vi "pwm servo.vi"(4 "Control 5":dbl, 6 "Control 4":dbl, 7 "Control 6":dbl, 9 "Control 3":dbl, 10 "Control 2":dbl, 11 "Control 1":dbl) -> ()   [LabVIEW 2019]
uses:
  <vilib>/myRIO/Instrument Drivers/Onboard IO/PWM/typedefs/PWM Reference.ctl
  <vilib>/myRIO/Common/Instrument Driver Framework/Utilities/typedefs/myRIO Generic Hardware Reference.ctl
  <vilib>/myRIO/Common/Instrument Driver Framework/Utilities/typedefs/Hardware Version Enum.ctl
  <vilib>/myRIO/Common/Instrument Driver Framework/Utilities/typedefs/myRIO v1.0 Reference.ctl
  <vilib>/myRIO/Common/Instrument Driver Framework/Utilities/typedefs/Generic FPGA Reference.ctl
  <vilib>/myRIO/Common/Instrument Driver Framework/myRIO v1.0/PWM/typedefs/PWM Channels Enum.ctl
  <vilib>/myRIO/Instrument Drivers/Onboard IO/PWM/typedefs/PWM Configuration.ctl
  <vilib>/userdefined/High Color/nirio_resource_hc.ctl
  <vilib>/myRIO/Common/Instrument Driver Framework/Utilities/vis/Is FPGA Ref Available.vi
  <vilib>/myRIO/Common/Instrument Driver Framework/myRIO v1.0/PWM/vis/myRIO v1.1 Open PWM.vi
  <vilib>/myRIO/Instrument Drivers/Onboard IO/PWM/vis/Set Duty Cycle and Frequency.vi
  <vilib>/myRIO/Common/Instrument Driver Framework/Utilities/vis/Validate Channels.vi
  <vilib>/myRIO/Common/Instrument Driver Framework/myRIO v1.0/PWM/vis/myRIO v1.0 Reserve PWM.vi
  <vilib>/myRIO/Common/Instrument Driver Framework/myRIO v1.0/PWM/vis/myRIO v1.0 Build MUX Configuration PWM.vi
  <vilib>/myRIO/Common/Instrument Driver Framework/myRIO v1.0/Resource Manager/vis/myRIO v1.0 Reserve Channel List.vi
  <vilib>/myRIO/Common/Instrument Driver Framework/myRIO v1.0/Resource Manager/vis/myRIO v1.0 Create Configuration List.vi
  <vilib>/myRIO/Common/Instrument Driver Framework/myRIO v1.0/Resource Manager/vis/myRIO v1.0 Reserve Channel.vi
  <vilib>/myRIO/Common/Instrument Driver Framework/myRIO v1.0/Resource Manager/vis/myRIO v1.0 Unreserve Channel.vi
  <vilib>/myRIO/Common/Instrument Driver Framework/myRIO v1.0/Resource Manager/vis/myRIO v1.0 Build Mutex Name.vi
  <vilib>/Utility/VariantDataType/GetNumericInfo.vi
  <vilib>/Utility/error.llb/Error Cluster From Error Code.vi
  <vilib>/myRIO/Common/Instrument Driver Framework/myRIO v1.0/myRIO v1.1 Open.vi
  <vilib>/myRIO/Common/Instrument Driver Framework/Utilities/vis/IO Manager.vi
  <vilib>/myRIO/Common/Instrument Driver Framework/Utilities/vis/Configuration Manager.vi
  <vilib>/myRIO/Common/Instrument Driver Framework/myRIO v1.0/Resource Manager/vis/myRIO v1.0 Configure IO.vi
  <vilib>/myRIO/Common/Instrument Driver Framework/myRIO v1.0/myRIO v1.0 Close.vi
  <vilib>/myRIO/Common/Instrument Driver Framework/myRIO v1.0/PWM/vis/myRIO v1.0 Write PWM.vi
  <vilib>/myRIO/Express VI/Onboard IO/PWM/PWM Express VI.xnode
  <vilib>/myRIO/Instrument Drivers/Onboard IO/PWM/vis/myRIO PWM Open.xnode
  <vilib>/myRIO/Instrument Drivers/Onboard IO/PWM/PWM.lvlib
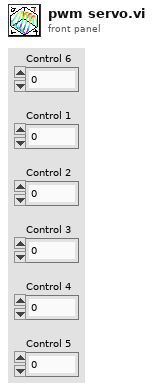
[diagram p1: front panel]
types:
  T1 = typedef "PWM.lvlib/PWM Reference.ctl" = cluster{"myRIO Reference":T2, "PWM Channels Enum":T6, "PWM Configuration":T7}
  T2 = typedef "myRIO Generic Hardware Reference.ctl" = cluster{"myRIO Model":T3, "myRIO Hardware Reference":T4}
  T3 = typedef "Hardware Version Enum.ctl" = enum16{"Unknown", "myRIO-1900", "myRIO-1950", "roboRIO", "NI ELVIS RIO CM", "ELVIS III"}
  T4 = typedef "myRIO v1.0 Reference.ctl" = cluster{"Generic FPGA Reference":T5, "Allow multiple opens":bool}
  T5 = typedef "Generic FPGA Reference.ctl" = refnum<k20>
  T6 = typedef "PWM Channels Enum.ctl" = enum16{"Not Connected", "C/PWM0", "C/PWM1", "A/PWM0", "A/PWM1", "A/PWM2", "A/PWM3", "A/PWM4", "A/PWM5", "A/PWM6", "A/PWM7", "A/PWM8", "A/PWM9", "A/PWM10", "A/PWM11", "A/PWM12", "A/PWM13", "A/PWM14", "A/PWM15", "A/PWM16", "A/PWM17", "A/PWM18", "A/PWM19", "B/PWM0", "B/PWM1", "B/PWM2", "B/PWM3", "B/PWM4", "B/PWM5", "B/PWM6", "B/PWM7", "B/PWM8", "B/PWM9", "B/PWM10", "B/PWM11", "B/PWM12", "B/PWM13", "B/PWM14", "B/PWM15", "B/PWM16", "B/PWM17", "B/PWM18", "B/PWM19", "PWM/PWM0", "PWM/PWM1", "PWM/PWM2", "PWM/PWM3", "PWM/PWM4", "PWM/PWM5", "PWM/PWM6", "PWM/PWM7", "PWM/PWM8", "PWM/PWM9"}
  T7 = typedef "PWM.lvlib/PWM Configuration.ctl" = cluster{"Frequency":dbl, "Duty Cycle":dbl}
  T8 = typedef "nirio_resource_hc.ctl" = tag
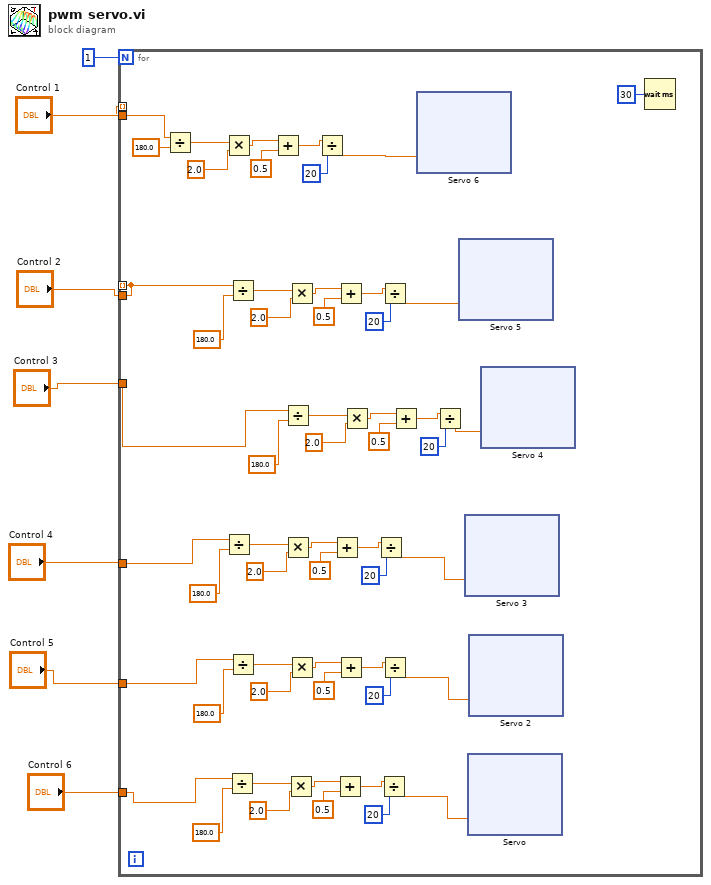
[diagram p0: block diagram]
diagram:
  n1 = for {
    N: 1 -> [_]
    tunnel: [w10] -> _ mode=indexing
    tunnel: [w9] -> _ mode=indexing
    tunnel: "Control 3" -> [w14]
    tunnel: "Control 4" -> [w13]
    tunnel: "Control 5" -> [w12]
    tunnel: "Control 1" -> [w10]
    tunnel: "Control 2" -> [w9]
    tunnel: "Control 6" -> [w8]
    n2 = Divide(x=w10, y=180.0) -> (x/y=w57:dbl)
    n3 = Multiply(x=w57, y=2.0) -> (x*y=w61:dbl)
    n4 = Divide(x=w13, y=180.0) -> (x/y=w33:dbl)
    n5 = Divide(x=w8, y=180.0) -> (x/y=w17:dbl)
    n6 = Divide(x=w9, y=180.0) -> (x/y=w49:dbl)
    n7 = Divide(x=w12, y=180.0) -> (x/y=w28:dbl)
    n8 = Add(x=w61, y=0.5) -> (x+y=w59:dbl)
    n9 = Divide(x=w14, y=180.0) -> (x/y=w44:dbl)
    n10 = Multiply(x=w33, y=2.0) -> (x*y=w37:dbl)
    n11 = Multiply(x=w17, y=2.0) -> (x*y=w21:dbl)
    n12 = Multiply(x=w49, y=2.0) -> (x*y=w53:dbl)
    n13 = Multiply(x=w28, y=2.0) -> (x*y=w24:dbl)
    n14 = Divide(x=w59, y=20) -> (x/y=w56:dbl)
    n15 = Add(x=w37, y=0.5) -> (x+y=w35:dbl)
    n16 = Add(x=w21, y=0.5) -> (x+y=w19:dbl)
    n17 = Add(x=w53, y=0.5) -> (x+y=w51:dbl)
    n18 = Add(x=w24, y=0.5) -> (x+y=w26:dbl)
    n19 = Multiply(x=w44, y=2.0) -> (x*y=w40:dbl)
    n20 = Divide(x=w35, y=20) -> (x/y=w32:dbl)
    n21 = Divide(x=w19, y=20) -> (x/y=w16:dbl)
    n22 = Divide(x=w51, y=20) -> (x/y=w48:dbl)
    n23 = Divide(x=w26, y=20) -> (x/y=w29:dbl)
    n24 = Add(x=w40, y=0.5) -> (x+y=w42:dbl)
    n25 = xnode "Servo 6"("Duty Cycle"=w56) -> ()  [unwired: 1 in, 1 out]
    n26 = Divide(x=w42, y=20) -> (x/y=w45:dbl)
    n27 = xnode "Servo 5"("Duty Cycle"=w48) -> ()  [unwired: 1 in, 1 out]
    n28 = xnode "Servo 3"("Duty Cycle"=w32) -> ()  [unwired: 1 in, 1 out]
    n29 = xnode "Servo"("Duty Cycle"=w16) -> ()  [unwired: 1 in, 1 out]
    n30 = xnode "Servo 2"("Duty Cycle"=w29) -> ()  [unwired: 1 in, 1 out]
    n31 = xnode "Servo 4"("Duty Cycle"=w45) -> ()  [unwired: 1 in, 1 out]
    n32 = Wait (ms)(milliseconds to wait=u32 30) -> ()  [unwired: 1 out]
  }
